vi "encodeTemperature.vi"(8 "error in (no error)":errorcluster, 10 "temperature":dbl, 11 "CameraNetworkServer in":refnum<class "CameraNetworkServer.lvclass">) -> (0 "error out":errorcluster, 2 "message":string, 3 "CameraNetworkServer out":refnum<class "CameraNetworkServer.lvclass">)   [LabVIEW 2011, in "Hardware.lvlib" / "HWControllers.lvlib" / "CameraNetworkServer.lvclass"]
uses:
  CameraNetworkServer.lvclass
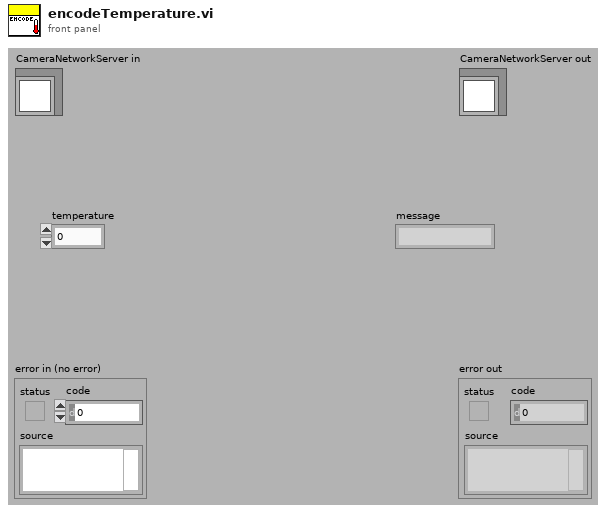
[diagram p1: front panel]
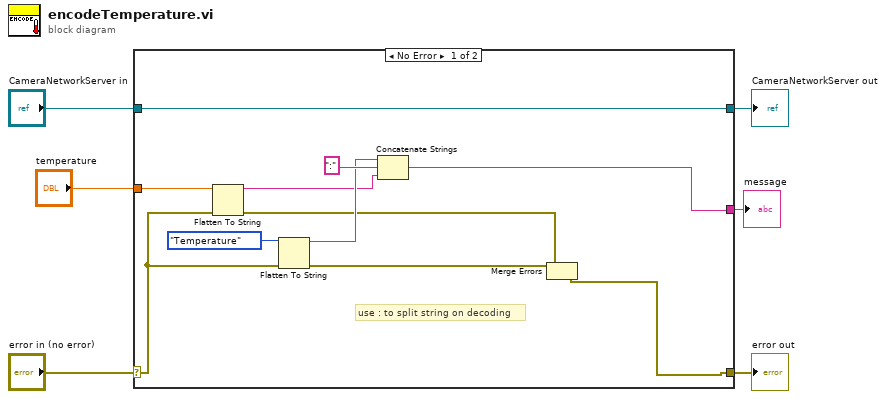
[diagram p0: block diagram]
diagram:
  n1 = case shown="No Error" "error in (no error)" {
    selector: "error in (no error)" -> [w9 w19]
    tunnel: [w7 w19] -> w5
    tunnel: [w17 w18] -> w3
    tunnel: "CameraNetworkServer in" -> [w17 w18]
    tunnel: "temperature" -> [w12 _]
    tunnel: [w10 _] -> w1
    frame No Error {
      # "use : to split string on decoding"
      n2 = Flatten To String(anything=w12, error in (no error)=w9) -> (data string=w11:string, error out=w8:errorcluster)  [unwired: 2 in, 1 out]
      n3 = Flatten To String(anything=enum16{"Temperature", "Image"}."Temperature", error in (no error)=w9) -> (data string=w13:string, error out=w15:errorcluster)  [unwired: 2 in, 1 out]
      n4 = Concatenate Strings(w13, ":", w11) -> (w10:string)
      n5 = Merge Errors(w8, w15) -> (w7:errorcluster)
    }
    frame Error {
    }
  }
  "error out" <- w5
  "CameraNetworkServer out" <- w3
  "message" <- w1
